vi "Present Data.vi"(8 "error in (no error)":errorcluster, 11 "List Seen Processes View Model In":refnum<class "Control View Model.lvclass">) -> (0 "error out":errorcluster, 2 "Message Data":variant, 3 "List Seen Processes View Model Out":refnum<class "Control View Model.lvclass">)   [LabVIEW 2020]
uses:
  Control View Model.lvclass
  Control View Model.lvclass/Control View Model.ctl
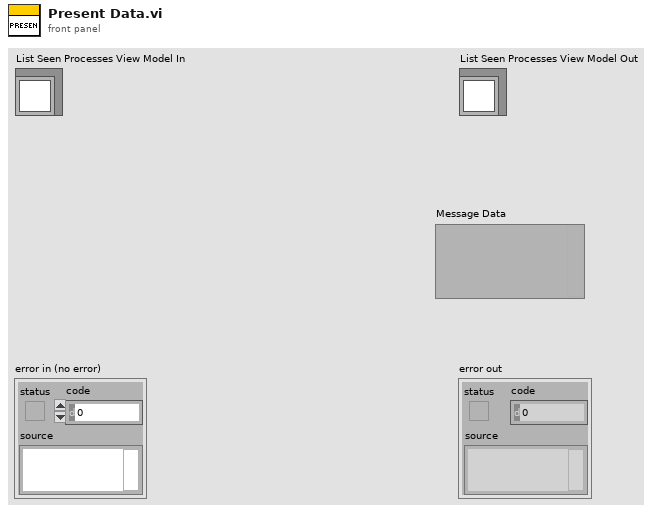
[diagram p1: front panel]
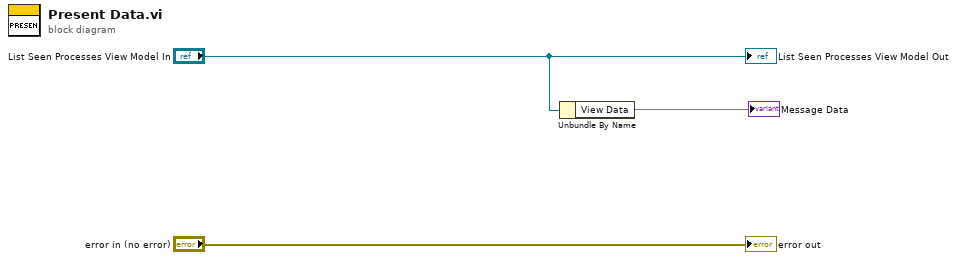
[diagram p0: block diagram]
diagram:
  n1 = Unbundle By Name("List Seen Processes View Model In") -> ("View Data"=→"Message Data")
  "error out" <- "error in (no error)"
  "List Seen Processes View Model Out" <- "List Seen Processes View Model In"
